vi "5802-filepath&name.vi"() -> ()   [LabVIEW 2020]
uses:
  <vilib>/Rock Robotics/Network Tables/NT Read String.vi
panel:
  out "path":path
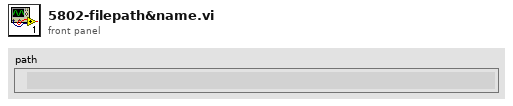
[diagram p1: front panel]
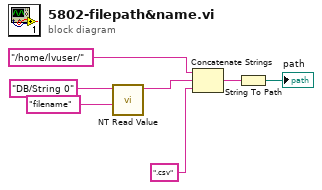
[diagram p0: block diagram]
diagram:
  n1 = call-poly <vilib>:"NT Read Value.vi"("Default Value"="filename", "Name"="DB/String 0") -> ("String"=w5:string)  [unwired: 8 in, 1 out]
  n2 = Concatenate Strings("/home/lvuser/", w5, ".csv") -> (w3:string)
  n3 = String To Path(string=w3) -> (path=→"path":path)
